vi "Text Description.vi"(11 "Message":refnum<class "Observer_RegisterForErrors.lvclass">) -> (2 "Description":string, 3 "Message":refnum<class "Observer_RegisterForErrors.lvclass">)   [LabVIEW 2011, in "Messenging.lvlib" / "Observer_RegisterForErrors.lvclass"]
uses:
  Observer_RegisterForErrors.lvclass
  ParentCommand/ObserverRegistryCommand.lvclass
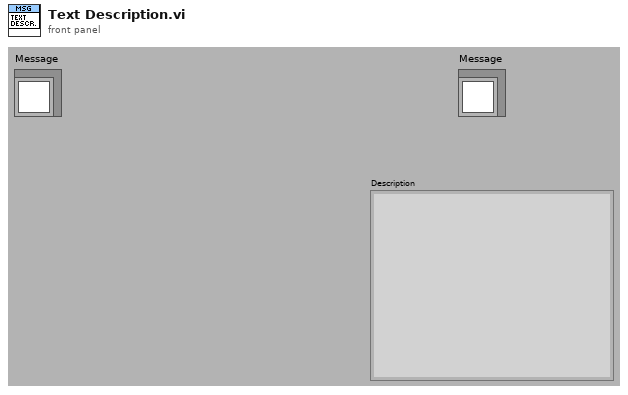
[diagram p1: front panel]
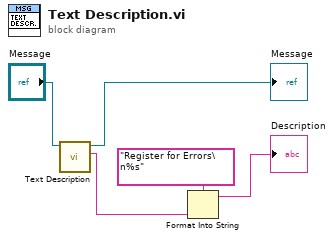
[diagram p0: block diagram]
diagram:
  n1 = call-parent "Text Description.vi"("Message"="Message") -> ("Description"=w2:string, "Message"=→"Message":refnum<class "Observer_RegisterForErrors.lvclass">)  [unwired: 9 out]
  n2 = Format Into String(format string="Register for Errors\n%s", w2) -> (resulting string=→"Description":string)  [unwired: 2 in, 1 out]
